vi "sort lookup table.vi"(8 "error in (no error)":errorcluster, 11 "lookup":variant) -> (0 "error out":errorcluster, 2 "tags by type":cluster{"indices":i32[], "names":string[]}[](array[cluster]), 3 "types":T1[](array[typedef]))   [LabVIEW 2013, in "tag bus.lvlib" / "data dictionary.lvclass"]
uses:
  data dictionary.lvclass
  tag/Data Type.ctl
  dictionary lookup value.ctl
  tag/tag descriptor.lvclass
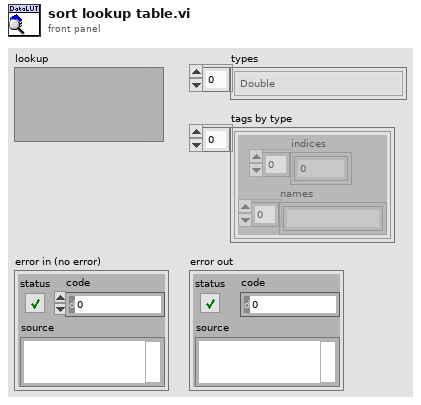
[diagram p1: front panel]
types:
  T1 = typedef "tag bus.lvlib/tag descriptor.lvclass/Data Type.ctl" = enum16{"Double", "Single", "I64", "I32", "I16", "I8", "U64", "U32", "U16", "U8", "Boolean", "String", "Array of Double", "Array of Single", "Array of I64", "Array of I32", "Array of I16", "Array of I8", "Array of U64", "Array of U32", "Array of U16", "Array of U8", "Array of Boolean", "Array of String"}
  T2 = typedef "tag bus.lvlib/data dictionary.lvclass/dictionary lookup value.ctl" = cluster{"data type":T1, "index":i32}
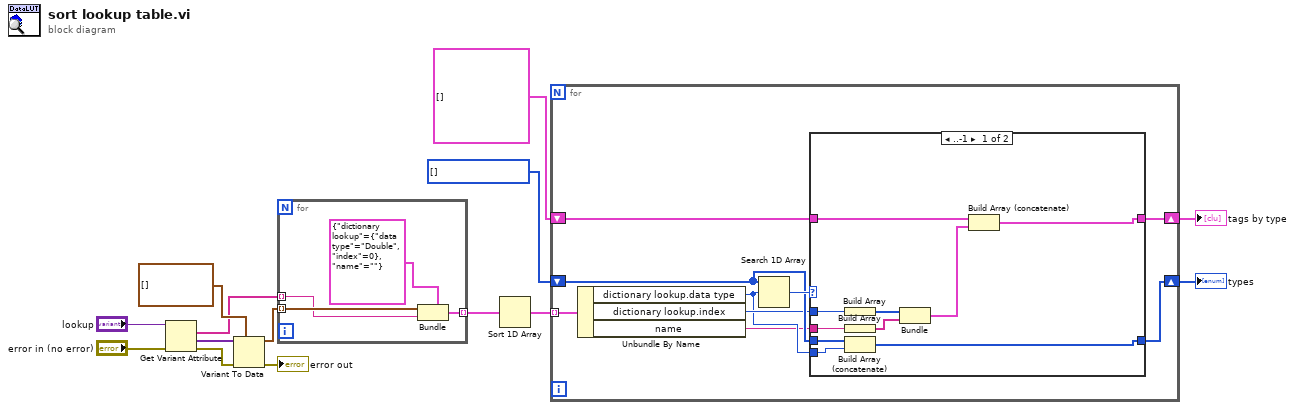
[diagram p0: block diagram]
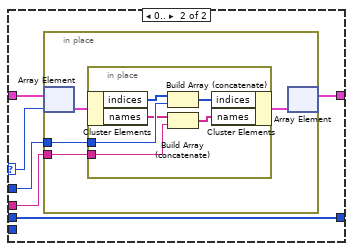
[diagram p2: hidden frame]
diagram:
  w12 = T1[] [] items=["Double", "Single", "I64", "I32", "I16", "I8", "U64", "U32", "U16", "U8", "Boolean", "String", "Array of Double", "Array of Single", "Array of I64", "Array of I32", "Array of I16", "Array of I8", "Array of U64", "Array of U32", "Array of U16", "Array of U8", "Array of Boolean", "Array of String"]
  n1 = Get Variant Attribute(Variant="lookup", error in="error in (no error)") -> (names=w3:string[], values=w10:variant[], error out=w6:errorcluster)  [unwired: 2 in, 1 out]
  n2 = Variant To Data(error in=w6, type=T2[] [], Variant=w10) -> (data=w4:T2[], error out=→"error out":errorcluster)
  n3 = for {
    tunnel: w4 -> [w18] mode=indexing
    tunnel: w3 -> [w17] mode=indexing
    tunnel: [w16] -> w2 mode=indexing
    n4 = Bundle(cluster=cluster{"dictionary lookup":T2, "name":string} {"dictionary lookup"={"data type"=enum."Double", "index"=0}, "name"=""}, "dictionary lookup"=w18, "name"=w17) -> (w16:cluster{"dictionary lookup":T2, "name":string})
  }
  n5 = Sort 1D Array(array=w2) -> (sorted array=w11:cluster{"dictionary lookup":T2, "name":string}[])
  n6 = for {
    tunnel: w11 -> [w27] mode=indexing
    shift-right: [w24] -> w14
    shift-left: w12 -> [w25]
    shift-right: [w22] -> w1
    shift-left: cluster{"indices":i32[], "names":string[]}[] [] -> [w23]
    n7 = Unbundle By Name(w27) -> ("dictionary lookup.data type"=w20:T1, "dictionary lookup.index"=w21:i32, "name"=w19:string)
    n8 = Search 1D Array(1D array=w25, element=w20) -> (index of element=w26:i32)  [unwired: 1 in]
    n9 = case shown="..-1" w26 {
      selector: w26 -> [_ w41]
      tunnel: w25 -> [w34 w43]
      tunnel: [w35 w43] -> w24
      tunnel: w23 -> [w37 w42]
      tunnel: [w36 w40] -> w22
      tunnel: w21 -> [w30 w39]
      tunnel: w20 -> [w33 _]
      tunnel: w19 -> [w28 w38]
      frame ..-1 {
        n10 = Build Array(w30) -> (w32:i32[])
        n11 = Build Array(w28) -> (w29:string[])
        n12 = Build Array (concatenate)(w34, w33) -> (w35:T1[])
        n13 = Bundle(w32, w29) -> (w31:cluster{i32[], string[]})  [unwired: 1 in]
        n14 = Build Array (concatenate)(w37, w31) -> (w36:cluster{"indices":i32[], "names":string[]}[])
      }
      frame 0.. {
        n15 = in-place {
          in-place-border: w39 -> [w45]
          in-place-border: w38 -> [w44]
          n16 = in-place-array #1(w42, w41) -> (w47:cluster{"indices":i32[], "names":string[]})
          n17 = in-place {
            in-place-border: w45 -> [w52]
            in-place-border: w44 -> [w48]
            n18 = in-place-cluster #2(w47) -> ("indices"=w53:i32[], "names"=w50:string[])
            n19 = Build Array (concatenate)(w53, w52) -> (w51:i32[])
            n20 = Build Array (concatenate)(w50, w48) -> (w49:string[])
            n21 = in-place-cluster #2("indices"=w51, "names"=w49) -> (w46:cluster{"indices":i32[], "names":string[]})
          }
          n22 = in-place-array #1(w46) -> (w40:cluster{"indices":i32[], "names":string[]}[])  [unwired: 1 out]
        }
      }
    }
  }
  "types" <- w14
  "tags by type" <- w1
